vi "file dialog cancel no error message.vi"(11 "prompt":string) -> (1 "cancelled":bool, 3 "path":path)   [LabVIEW 2023]
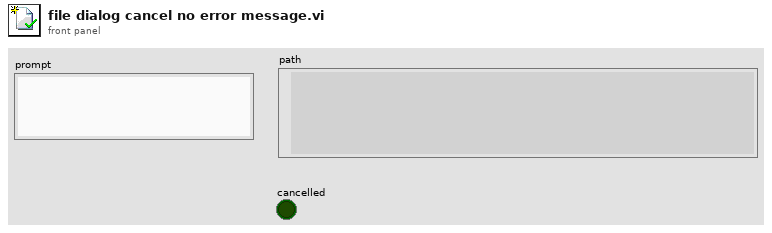
[diagram p1: front panel]
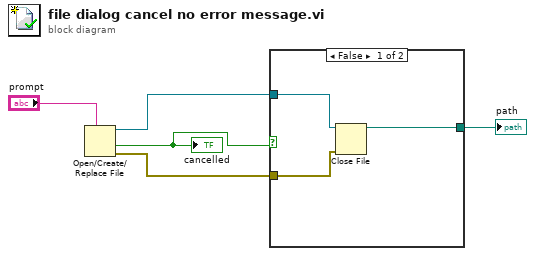
[diagram p0: block diagram]
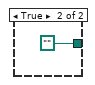
[diagram p2: hidden frame]
diagram:
  n1 = Open/Create/Replace File(prompt="prompt") -> (refnum out=w5:refnum<file>, cancelled=w3:bool, error out=w4:errorcluster)  [unwired: 5 in]
  "cancelled" <- w3
  n2 = case shown="False" w3 {
    tunnel: w5 -> [w8 _]
    tunnel: w4 -> [w7 _]
    tunnel: [w6 path ""] -> w1
    frame False {
      n3 = Close File(refnum=w8, error in=w7) -> (path=w6:path)  [unwired: 1 out]
    }
    frame True {
    }
  }
  "path" <- w1
